vi "Frame Process.vi"(8 "error in (no error)":errorcluster, 10 "Video Frame In":refnum<class "Video Frame.lvclass">, 11 "Video Processor in":refnum<class "Video Processor.lvclass">) -> (0 "error out":errorcluster, 3 "Video Processor out":refnum<class "Video Processor.lvclass">)   [LabVIEW 2018, in "Video Processor.lvclass"]
uses:
  Video Processor.lvclass
  Video Frame/Video Frame.lvclass
  Video Processor.lvclass/Video Processor.ctl
  6936c895-b0a3-4e2c-9892-7cf1b7938e16.vi
  5fbe6361-8a29-4a31-af02-72406432bcc9.vi
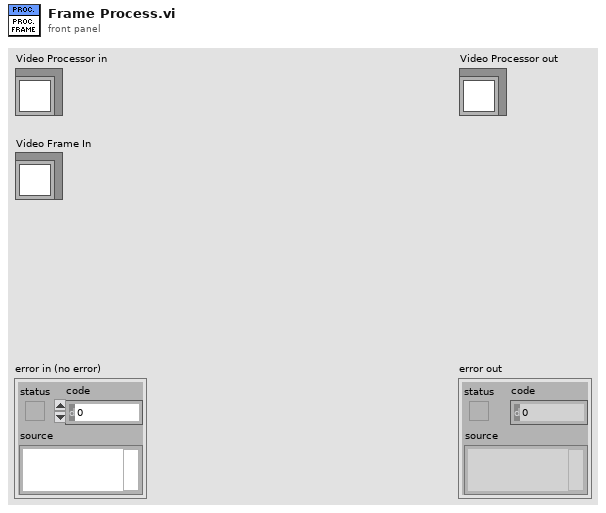
[diagram p1: front panel]
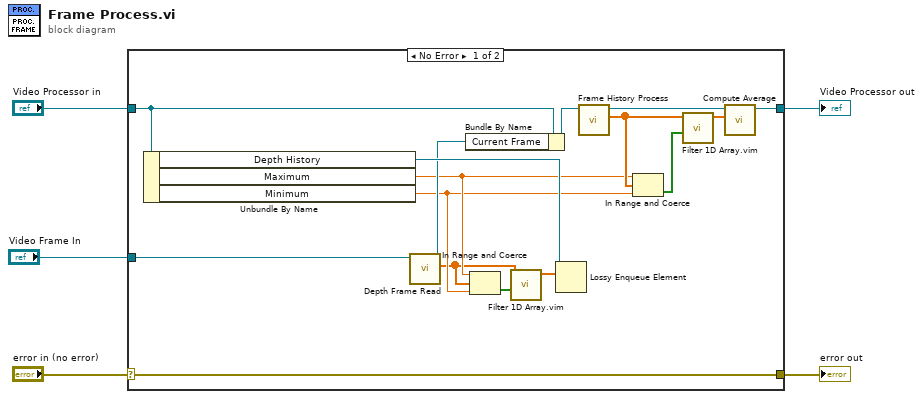
[diagram p0: block diagram]
diagram:
  n1 = case shown="No Error" "error in (no error)" {
    selector: "error in (no error)" -> [w21 w23]
    tunnel: [w21 w23] -> w4
    tunnel: [w16 w22] -> w2
    tunnel: "Video Processor in" -> [w7 w22]
    tunnel: "Video Frame In" -> [w6 _]
    frame No Error {
      n2 = Unbundle By Name(w7) -> ("Depth History"=w20:refnum<queue>, "Maximum"=w12:dbl, "Minimum"=w11:dbl)
      n3 = call-dynamic "Depth Frame Read.vi"("Video Frame in"=w6) -> ("Depth Values"=w10:dbl[], "Video Frame out"=w19:refnum<class "Video Frame.lvclass">)  [unwired: 6 in, 3 out]
      n4 = Bundle By Name(cluster=w7, "Current Frame"=w19) -> (w18:refnum<class "Video Processor.lvclass">)
      n5 = In Range and Coerce(upper limit=w12, x=w10, lower limit=w11) -> (In Range?=w9:bool[])  [unwired: 1 out]
      n6 = call "Filter 1D Array.vim"("Boolean Filter"=w9, "Array"=w10) -> ("Array Out"=w8:dbl[])  [unwired: 9 in]
      n7 = Lossy Enqueue Element(queue=w20, element=w8) -> ()  [unwired: 1 in, 4 out]
      n8 = call-dynamic "Frame History Process.vi"("Video Processor in"=w18) -> ("Depth Values Out"=w14:dbl[], "Video Processor out"=w17:refnum<class "Video Processor.lvclass">)  [unwired: 8 in, 1 out]
      n9 = In Range and Coerce(upper limit=w12, x=w14, lower limit=w11) -> (In Range?=w13:bool[])  [unwired: 1 out]
      n10 = call "Filter 1D Array.vim"("Boolean Filter"=w13, "Array"=w14) -> ("Array Out"=w15:dbl[])  [unwired: 9 in]
      n11 = call-dynamic "Compute Average.vi"("Data"=w15, "Video Processor in"=w17) -> ("Video Processor out"=w16:refnum<class "Video Processor.lvclass">)  [unwired: 8 in, 1 out]
    }
    frame Error {
    }
  }
  "error out" <- w4
  "Video Processor out" <- w2
